vi "LoadApp.vi"() -> (0 "error out":errorcluster)   [LabVIEW 2024, in "MFActor.lvlib" / "MFActor.lvclass"]
uses:
  MFActor.lvclass
  C:/Program Files (x86)/National Instruments/LabVIEW 2024/vi.lib/ActorFramework/Actor/Actor.lvclass
  DeviceAlias.ctl
  NestedActorName.ctl
  MFActor.lvclass/MFActor.ctl
  <vilib>/ActorFramework/Actor/Actor.lvclass
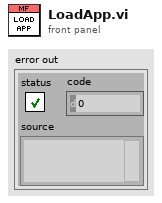
[diagram p1: front panel]
types:
  T1 = typedef "NestedActorName.ctl" = enum16{"None", "4503#0", "4503#1", "AIO#0", "AIO#1", "DIO", "PID", "TCPIP", "TestAngle", "TestFixPt", "TestMultiPt", "TestSinWave", "PW3390"}
  T2 = typedef "DeviceAlias.ctl" = enum16{"TQM0", "TQM1", "PM", "THERMO", "DC POWER"}
  T3 = cluster{"Period(sec)":dbl, "WaveCrest":dbl, "WaveTrough":dbl}
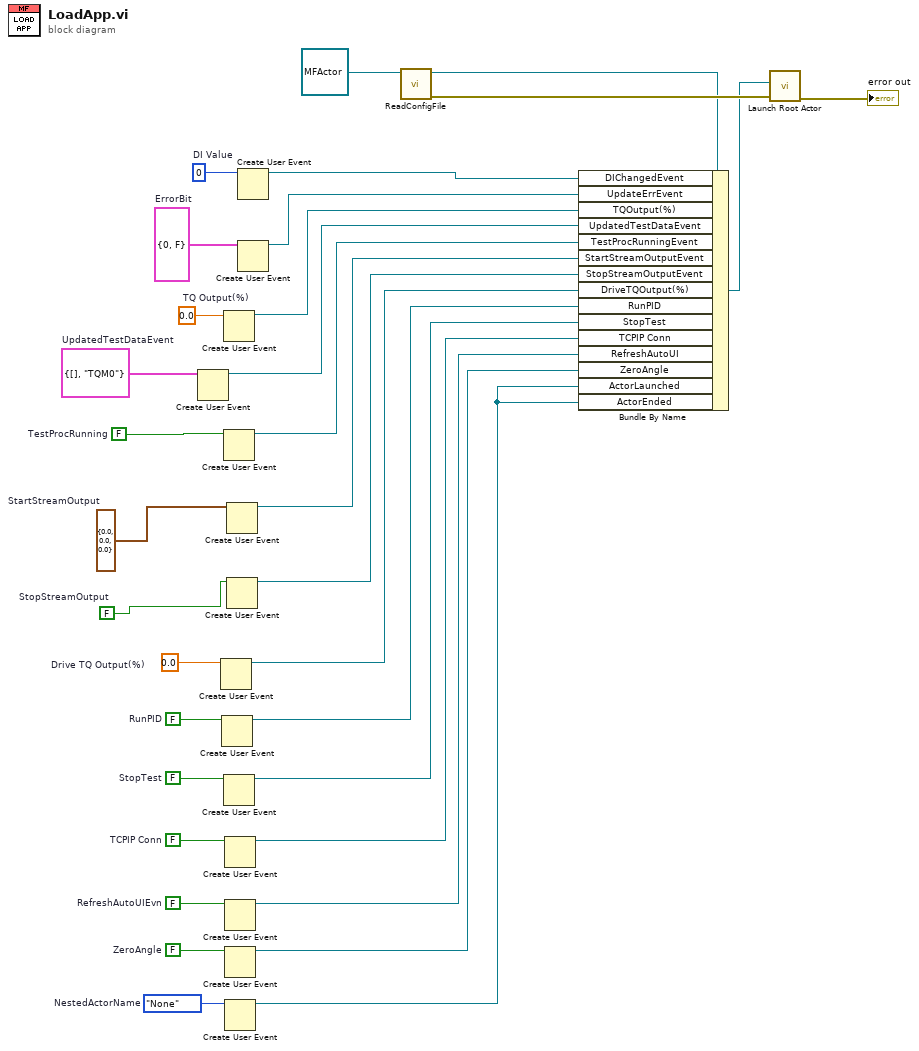
[diagram p0: block diagram]
diagram:
  w2 = NestedActorName."None"  # NestedActorName
  w4 = cluster{"TestDataDBL":dbl[], "Device":T2} {"TestDataDBL"=[], "Device"=enum."TQM0"}  # UpdatedTestDataEvent
  w6 = FALSE  # ZeroAngle
  w8 = FALSE  # RefreshAutoUIEvn
  w10 = FALSE  # TCPIP Conn
  w12 = FALSE  # StopTest
  w14 = FALSE  # RunPID
  w16 = 0.0  # Drive TQ Output(%)
  w19 = FALSE  # StopStreamOutput
  w20 = T3 {"Period(sec)"=0.0, "WaveCrest"=0.0, "WaveTrough"=0.0}  # StartStreamOutput
  w22 = FALSE  # TestProcRunning
  w24 = 0.0  # TQ Output(%)
  w26 = cluster{"Bit":i32, "Error":bool} {"Bit"=0, "Error"=FALSE}  # ErrorBit
  w30 = u32 0  # DI Value
  n1 = Create User Event(user event datatype=w4) -> (user event=w3:refnum<user-event>)  [unwired: 1 in, 1 out]
  n2 = Create User Event(user event datatype=w16) -> (user event=w15:refnum<user-event>)  [unwired: 1 in, 1 out]
  n3 = Create User Event(user event datatype=w14) -> (user event=w13:refnum<user-event>)  [unwired: 1 in, 1 out]
  n4 = Create User Event(user event datatype=w24) -> (user event=w23:refnum<user-event>)  [unwired: 1 in, 1 out]
  n5 = Create User Event(user event datatype=w22) -> (user event=w21:refnum<user-event>)  [unwired: 1 in, 1 out]
  n6 = Create User Event(user event datatype=w12) -> (user event=w11:refnum<user-event>)  [unwired: 1 in, 1 out]
  n7 = Create User Event(user event datatype=w10) -> (user event=w9:refnum<user-event>)  [unwired: 1 in, 1 out]
  n8 = Create User Event(user event datatype=w8) -> (user event=w7:refnum<user-event>)  [unwired: 1 in, 1 out]
  n9 = Create User Event(user event datatype=w6) -> (user event=w5:refnum<user-event>)  [unwired: 1 in, 1 out]
  n10 = Create User Event(user event datatype=w2) -> (user event=w1:refnum<user-event>)  [unwired: 1 in, 1 out]
  n11 = Create User Event(user event datatype=w20) -> (user event=w18:refnum<user-event>)  [unwired: 1 in, 1 out]
  n12 = Create User Event(user event datatype=w19) -> (user event=w17:refnum<user-event>)  [unwired: 1 in, 1 out]
  n13 = Create User Event(user event datatype=w30) -> (user event=w28:refnum<user-event>)  [unwired: 1 in, 1 out]
  n14 = Create User Event(user event datatype=w26) -> (user event=w25:refnum<user-event>)  [unwired: 1 in, 1 out]
  n15 = call "ReadConfigFile.vi"("MFActor in"=refnum<class "MFActor.lvclass"> refnum ("MFActor.lvlib:MFActor.lvclass")) -> ("error out"=w31:errorcluster, "MFActor out"=w29:refnum<class "MFActor.lvclass">)  [unwired: 9 in]
  n16 = Bundle By Name(cluster=w29, "DIChangedEvent"=w28, "UpdateErrEvent"=w25, "TQOutput(%)"=w23, "UpdatedTestDataEvent"=w3, "TestProcRunningEvent"=w21, "StartStreamOutputEvent"=w18, "StopStreamOutputEvent"=w17, "DriveTQOutput(%)"=w15, "RunPID"=w13, "StopTest"=w11, "TCPIP Conn"=w9, "RefreshAutoUI"=w7, "ZeroAngle"=w5, "ActorLaunched"=w1, "ActorEnded"=w1) -> (w27:refnum<class "MFActor.lvclass">)
  n17 = call <vilib>:"Launch Root Actor.vi"("error in (no error)"=w31, "Actor"=w27) -> ("error out"=→"error out":errorcluster)  [unwired: 8 in, 1 out]
